vi "LVClass_Image ctor from Image NarrowFilter.vi"(0 "Image( const)":refnum<class "Image.lvclass">, 5 "Image":refnum<class "Image.lvclass">, 7 "config_file_path":path, 11 "error in (no error)":errorcluster) -> (4 "Image (new)":refnum<class "Image.lvclass">, 6 "Image (dup)":refnum<class "Image.lvclass">, 15 "error out":errorcluster)   [LabVIEW 2020, in "Image.lvclass"]
doc: "Inplace subtraction : ImageA = ImageA \\- ImageB. Images must have the same\nsize, channels count and bits depth.\n\n--------------------------------------------------------------------------------\n\n<B>ImageAIn </B> : Image object.\n<B>ImageAOut </B> : Image object.\n<B>ImageB </B> : Image object.\n<B>ErrorIn </B> : Error\n<B>ErrorOut </B> : Error\n\n--------------------------------------------------------------------------------"
uses:
  Image.lvclass
  Handle creation.ctl
  Image.lvclass/Image.ctl
  LVClass_Image Read Image.vi
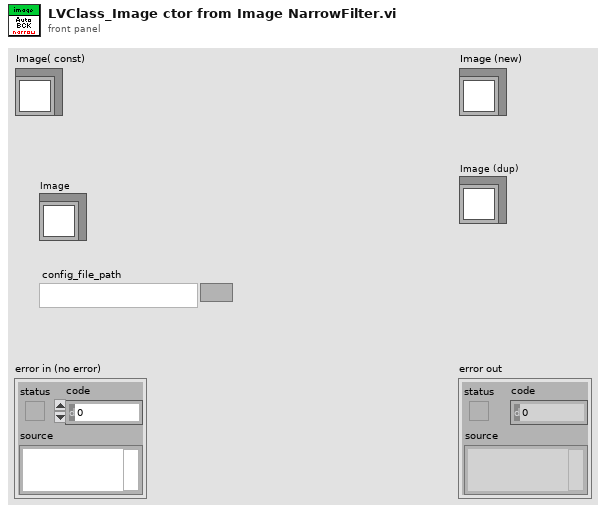
[diagram p1: front panel]
types:
  T1 = typedef "Handle creation.ctl" = enum16{"By ctor", "By write function"}
  T2 = typedef "Struct_Image.ctl" = cluster{"Image_Handler":T3, "Number of bits":T4, "ImageSize":T5}
  T3 = typedef "ClassID.ctl" = i64
  T4 = typedef "Data alignment enum.ctl" = enum16{"8", "16", "32"}
  T5 = typedef "Point2D.ctl" = cluster{"X":u32, "Y":u32}
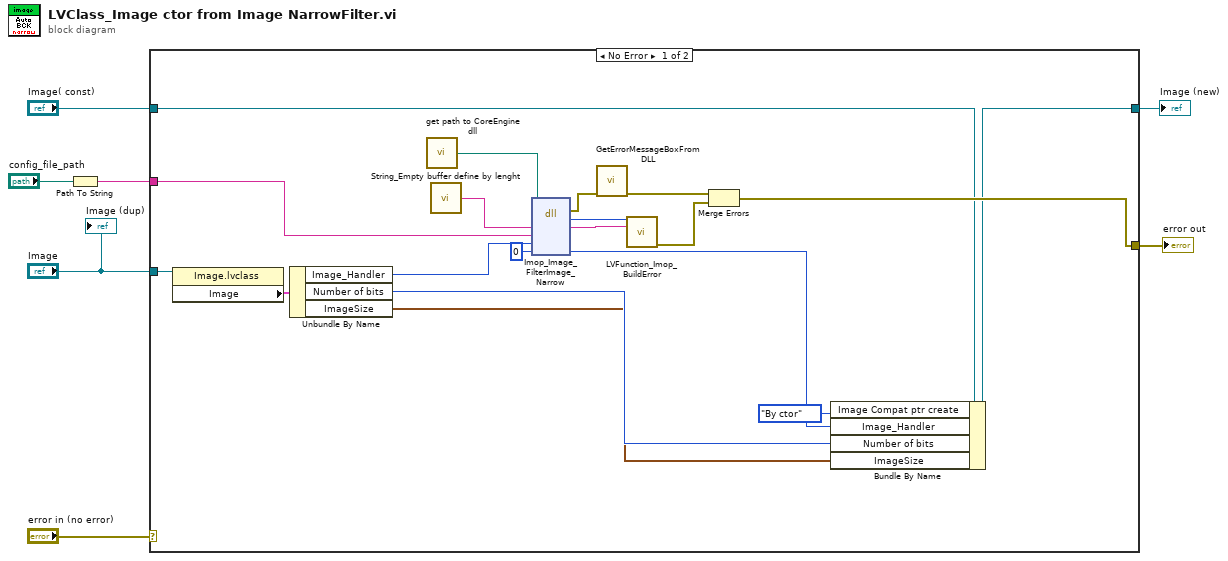
[diagram p0: block diagram]
diagram:
  n1 = Path To String(path="config_file_path") -> (string=w1:string)
  n2 = case shown="No Error" "error in (no error)" {
    selector: "error in (no error)" -> [_ w28]
    tunnel: [w19 w28] -> w6
    tunnel: [w10 w27] -> w5
    tunnel: "Image( const)" -> [w9 w27]
    tunnel: "Image" -> [w13 _]
    tunnel: w1 -> [w8 _]
    frame No Error {
      n3 = property class="Image.lvclass"(reference=w13) -> ("Image"=w16:T2)  [unwired: 1 in, 2 out]
      n4 = Unbundle By Name(w16) -> ("Image_Handler"=w12:T3, "Number of bits"=w15:T4, "ImageSize"=w14:T5)
      n5 = call "get path to CoreEngine dll.vi"() -> ("path to c_interface_vc100.dll"=w23:path)  [unwired: 12 in, 3 out]
      n6 = call "String_Empty buffer define by lenght.vi"() -> ("Empty buffer"=w26:string)  [unwired: 1 in]
      n7 = dll-call lib="D:/2_trunk/Soft_haso/ImOpCoreEngine4_LV2011/DLLs/ImopEngine4_vc100.dll" fn="Imop_Image_FilterImage_Narrow"(path in=w23, "message"=w26, "config_file_path"=w8, "Image"=w12, "NewImage"=i64 0) -> (error out=w22:errorcluster, "return type"=w25:i32, "message"=w24:string, "NewImage"=w11:i64)  [unwired: 4 in, 1 out]
      n8 = call "GetErrorMessageBoxFromDLL.vi"("error IN"=w22) -> ("error OUT"=w21:errorcluster)  [unwired: 10 in]
      n9 = call "LVFunction_Imop_BuildError.vi"("code"=w25, "String to Prepend to source (\"\")"=w24) -> ("error out"=w20:errorcluster)  [unwired: 13 in]
      n10 = Merge Errors(w21, w20) -> (w19:errorcluster)
      n11 = Bundle By Name(cluster=w9, "Image Compat ptr create"=Handle_creation."By ctor", "Image_Handler"=w11, "Number of bits"=w15, "ImageSize"=w14) -> (w10:refnum<class "Image.lvclass">)
    }
    frame Error {
    }
  }
  "error out" <- w6
  "Image (new)" <- w5
  "Image (dup)" <- "Image"
